vi "ReadWrite Channels.vi"(4 "ScheduledSDI":bool, 6 "Iteration":i32, 7 "Mode":T13, 8 "error in (no error)":errorcluster, 10 "FIFOs In":T14, 11 "Channels In":T1[](array[typedef]) {"Labels Settings"."Label" format="%.0o"}) -> (0 "error out":errorcluster, 2 "FIFOs Out":T14, 3 "Channels Out":T1[](array[typedef]) {"Labels Settings"."Label" format="%.0o"})   [LabVIEW 2015, in "AIT 429 Engine.lvlib"]
uses:
  AIT 429 Engine.lvlib
  RT Controls/FIFO.ctl
  RT Controls/ReadWrite Selector.ctl
  RT Controls/RT HW Channel.ctl
  RT Controls/RT Label Settings.ctl
  Shared/Controls and Global/Label.ctl
  Shared/Controls and Global/transferPeriod.ctl
  RT Controls/Driver Data.ctl
  RT Controls/RT Word Settings.ctl
  <vilib>/NI Veristand/Custom Device API/Block Data Reference.ctl
  <vilib>/NI Veristand/Custom Device API/Data Reference.ctl
  RT Controls/RT Param Setting.ctl
  Shared/Controls and Global/Start Bit.ctl
  Shared/Controls and Global/Number of Bits.ctl
  Shared/Controls and Global/TransferType.ctl
  Write outgoing label data.vi
  Read incoming label data.vi
  Read Parameter VS Channels.vi
  Update Parameter VS Channels.vi
  Double to selected bits.vi
  Shared/Word to double.vi
  <vilib>/NI Veristand/Custom Device API/NI VeriStand - Get Channel Values by Block Data Reference.vi
  <vilib>/NI Veristand/Custom Device API/NI VeriStand - Set Channel Values by Block Data Reference.vi
  <vilib>/NI Veristand/Custom Device API/Global Data Refs.vi
  <instrlib>/AIT 429/Public/Tx/Data/AIT 429 Set Acyclic Transfer Data.vi
  <instrlib>/AIT 429/Public/Tx/Data/AIT 429 Get Acyclic Transfer Data.vi
  <instrlib>/AIT 429/Public/Tx/Data/AIT 429 Set Block Transfer Data.vi
  <instrlib>/AIT 429/Public/Tx/Data/AIT 429 Get Block Transfer Data.vi
  <instrlib>/AIT 429/Public/Tx/Data/AIT 429 Set Scheduled Label Data.vi
  <instrlib>/AIT 429/Public/Tx/Data/AIT 429 Get Scheduled Label Data.vi
  <instrlib>/AIT 429/AIT 429.lvlib
  <userlib>/ARINC-429/Owl429.lvlib
  Shared/AIT 429 Shared.lvlib
  <vilib>/NI Veristand/Custom Device API/Custom Device API.lvlib
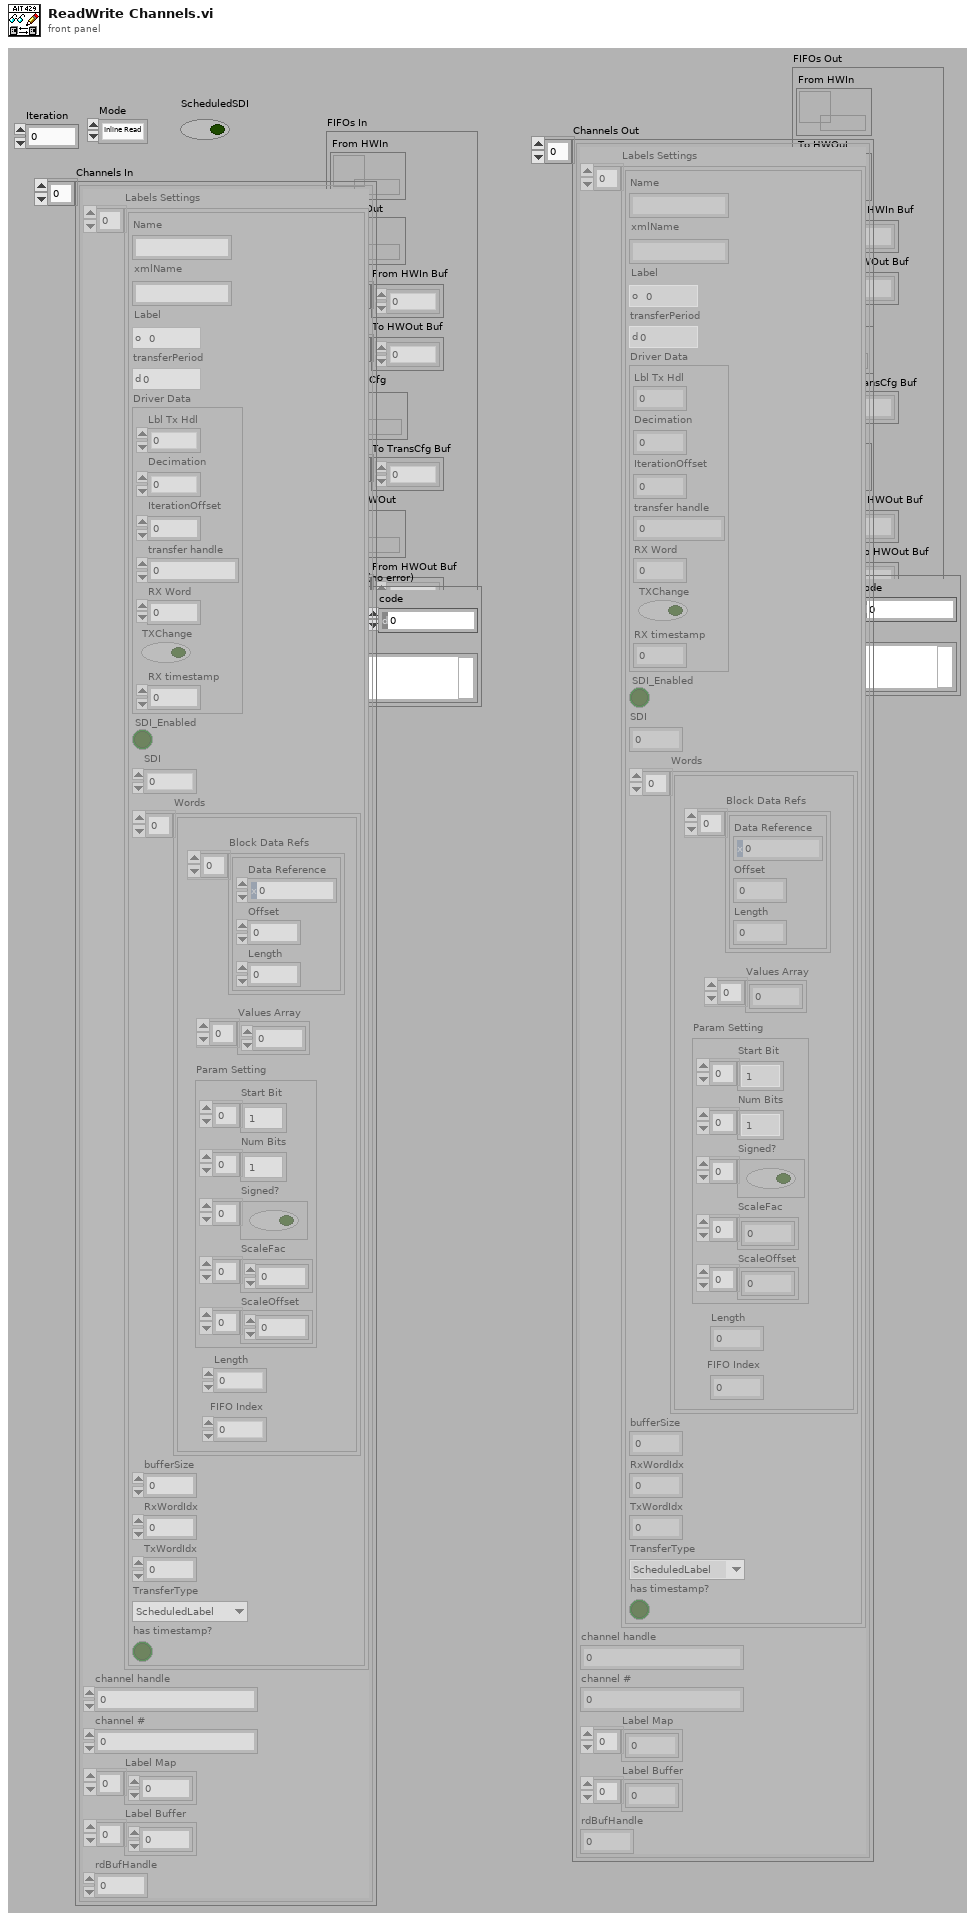
[diagram p1: front panel]
types:
  T1 = typedef "AIT 429 Engine.lvlib/RT HW Channel.ctl" = cluster{"Labels Settings":T2[], "channel handle":u32, "channel #":u16, "Label Map":i32[], "Label Buffer":u32[], "rdBufHandle":u32}
  T2 = typedef "AIT 429 Engine.lvlib/RT Label Settings.ctl" = cluster{"Name":string, "xmlName":string, "Label":T3, "transferPeriod":T4, "Driver Data":T5, "SDI_Enabled":bool, "SDI":u8, "Words":T6[], "bufferSize":u32, "RxWordIdx":i32, "TxWordIdx":i32, "TransferType":T12, "has timestamp?":bool}
  T3 = typedef "AIT 429 Shared.lvlib/Label.ctl" = u8
  T4 = typedef "AIT 429 Shared.lvlib/transferPeriod.ctl" = u32
  T5 = typedef "AIT 429 Engine.lvlib/Driver Data.ctl" = cluster{"Lbl Tx Hdl":u32, "Decimation":i32, "IterationOffset":i32, "transfer handle":u32, "RX Word":u32, "TXChange":bool, "RX timestamp":dbl}
  T6 = typedef "AIT 429 Engine.lvlib/RT Word Settings.ctl" = cluster{"Block Data Refs":T7[], "Values Array":dbl[], "Length":i32, "FIFO Index":i32, "Param Setting":T9}
  T7 = typedef "Custom Device API.lvlib/Block Data Reference.ctl" = cluster{"Data Reference":T8, "Offset":u64, "Length":u64}
  T8 = typedef "Custom Device API.lvlib/Data Reference.ctl" = i32
  T9 = typedef "AIT 429 Engine.lvlib/RT Param Setting.ctl" = cluster{"Start Bit":T10[], "Num Bits":T11[], "Signed?":bool[], "ScaleFac":dbl[], "ScaleOffset":dbl[]}
  T10 = typedef "AIT 429 Shared.lvlib/Start Bit.ctl" = i32
  T11 = typedef "AIT 429 Shared.lvlib/Number of Bits.ctl" = i32
  T12 = typedef "AIT 429 Shared.lvlib/TransferType.ctl" = enum16{"ScheduledLabel", "Acyclic", "Block", "Strobe"}
  T13 = typedef "AIT 429 Engine.lvlib/ReadWrite Selector.ctl" = enum16{"Inline Read", "Inline Write", "Async HWIn", "Async HWOut"}
  T14 = typedef "AIT 429 Engine.lvlib/FIFO.ctl" = cluster{"From HWIn":refnum<k33>, "To HWOut":refnum<k33>, "From HWIn Buf":dbl[], "To HWOut Buf":dbl[], "To TansCfg":refnum<k33>, "To TransCfg Buf":dbl[], "From HWOut":refnum<k33>, "From HWOut Buf":dbl[], "Old To HWOut Buf":dbl[]}
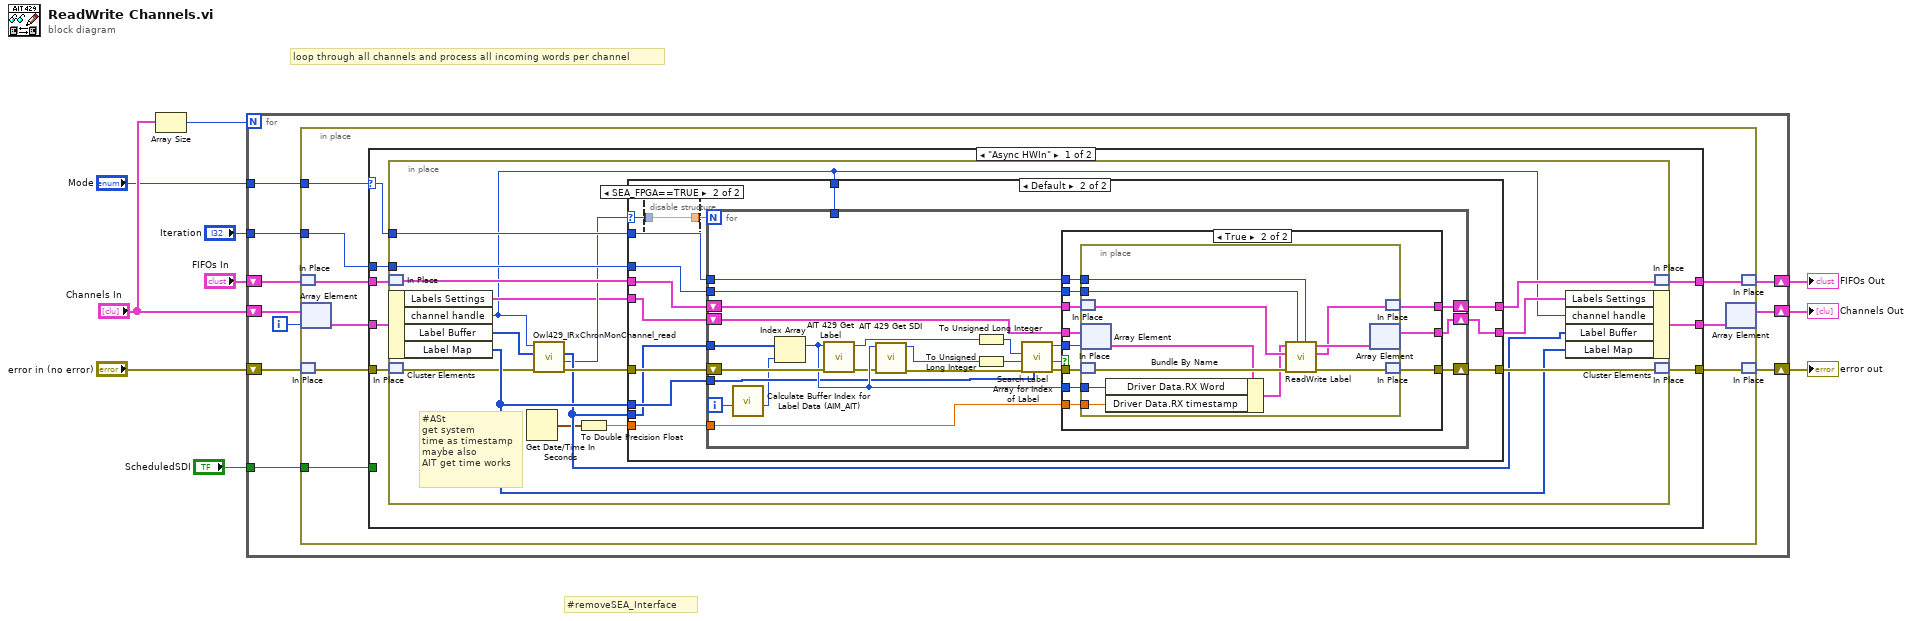
[diagram p0: block diagram]
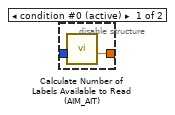
[diagram p3: hidden frame]
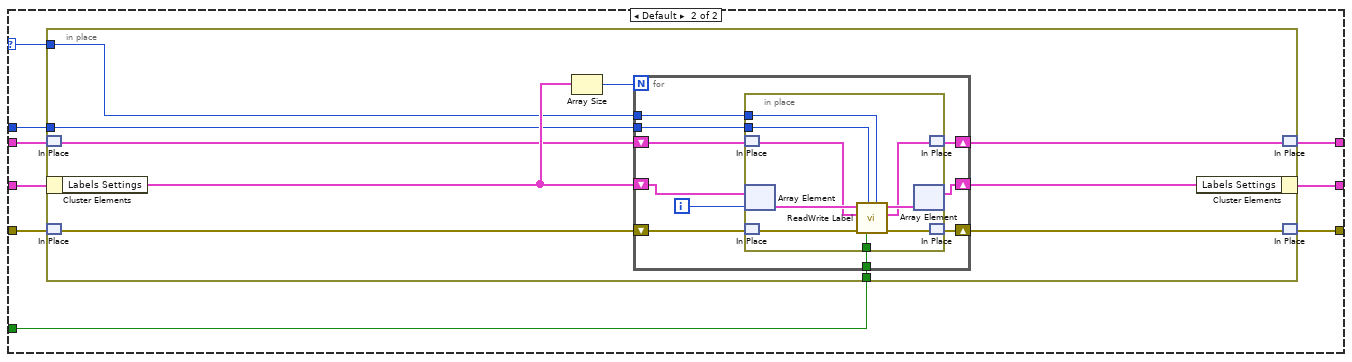
[diagram p5: hidden frame]
diagram:
  # "#removeSEA_Interface"
  # "loop through all channels and process all incoming words per channel"
  n1 = Array Size(array="Channels In") -> (size(s)=w5:i32)
  n2 = for {
    N: w5 -> [_]
    shift-right: [w17] -> w8
    shift-left: "error in (no error)" -> [w18]
    tunnel: "Mode" -> [w16]
    tunnel: "Iteration" -> [w13]
    shift-right: [w19] -> w7
    shift-left: "Channels In" -> [w20]
    shift-right: [w14] -> w10
    shift-left: "FIFOs In" -> [w15]
    tunnel: "ScheduledSDI" -> [w12]
    i -> [w11]
    n3 = in-place {
      in-place-border: w16 -> [w22]
      in-place-border: w13 -> [w23]
      in-place-border: w12 -> [w21]
      n4 = in-place-match #1(w15) -> (w25:T14)
      n5 = in-place-array #2(w20, w11) -> (w29:T1)
      n6 = in-place-match #3(w18) -> (w27:errorcluster)
      n7 = case shown="\"Async HWIn\"" w22 {
        selector: w22 -> [w30 w123]
        tunnel: w29 -> [w37 w130]
        tunnel: [w36 w129] -> w28
        tunnel: w27 -> [w35 w128]
        tunnel: [w34 w127] -> w26
        tunnel: w25 -> [w33 w126]
        tunnel: [w32 w125] -> w24
        tunnel: w23 -> [w31 w124]
        tunnel: w21 -> [_ w122]
        frame "Async HWIn" {
          n8 = in-place {
            in-place-border: w30 -> [w51]
            in-place-border: w31 -> [w49]
            # "#ASt\nget system\ntime as timestamp\nmaybe also\nAIT get time works"
            n9 = in-place-match #4(w33) -> (w48:T14)
            n10 = in-place-cluster #5(w37) -> ("Labels Settings"=w41:T2[], "channel handle"=w38:u32, "Label Buffer"=w42:u32[], "Label Map"=w47:i32[])
            n11 = in-place-match #6(w35) -> (w45:errorcluster)
            n12 = Get Date/Time In Seconds() -> (seconds since 1Jan1904=w40:timestamp)
            n13 = call <userlib>:"Owl429_IRxChronMonChannel_read.vi"("error in (no error)"=w45, "data buffer"=w42, "channel handle"=w38) -> ("error out"=w46:errorcluster, "word count"=w43:u32, "data buffer"=w44:u32[])  [unwired: 5 in, 1 out]
            n14 = To Double Precision Float(number=w40) -> (double precision float=w39:dbl)
            n15 = case shown="Default" w43 {
              selector: w43 -> [_ w59]
              tunnel: w41 -> [w55 w70]
              tunnel: [w55 w69] -> w53
              tunnel: [w56 w68] -> w52
              tunnel: w51 -> [_ w67]
              tunnel: [w54 w66] -> w50
              tunnel: w49 -> [_ w65]
              tunnel: w48 -> [w54 w64]
              tunnel: w47 -> [_ w63]
              tunnel: w46 -> [w56 w62]
              tunnel: w44 -> [_ w61]
              tunnel: w39 -> [_ w58]
              tunnel: w38 -> [_ w57]
              frame 0 {
              }
              frame Default {
                n16 = disable-structure shown="SEA_FPGA==TRUE" {
                  disable-tunnel: [w72 w73] -> w60
                  disable-tunnel: w59 -> [w71 w73]
                  frame condition #0 (active) {
                    n17 = call "Calculate Number of Labels Available to Read (AIM_AIT).vi"("entry count"=w71) -> ("# of labels available"=w72:dbl)  [unwired: 10 in]
                  }
                  frame condition #1 {
                  }
                }
                n18 = for {
                  N: w60 -> [_]
                  shift-right: [w95] -> w68
                  shift-left: w62 -> [w90]
                  tunnel: w67 -> [w94]
                  tunnel: w65 -> [w91]
                  tunnel: w61 -> [w86]
                  shift-right: [w92] -> w66
                  shift-left: w64 -> [w93]
                  shift-right: [w96] -> w69
                  shift-left: w70 -> [w89]
                  tunnel: w63 -> [w76]
                  tunnel: w58 -> [w77]
                  tunnel: w57 -> [_]
                  i -> [w84]
                  n19 = call "Calculate Buffer Index for Label Data (AIM_AIT).vi"("Iteration"=w84) -> ("Buffer index"=w75:u32)  [unwired: 10 in]
                  n20 = Index Array(array=w86, index=w75) -> (element=w80:u32)
                  n21 = call <instrlib>:"AIT 429 Get Label.vi"("error in (no error)"=w90, "word"=w80) -> ("error out"=w74:errorcluster, "label"=w81:u8)  [unwired: 8 in]
                  n22 = call <instrlib>:"AIT 429 Get SDI.vi"("error in (no error)"=w74, "word"=w80) -> ("error out"=w82:errorcluster, "sdi"=w83:u8)  [unwired: 8 in]
                  n23 = To Unsigned Long Integer(number=w81) -> (unsigned 32bit integer=w79:u32)
                  n24 = To Unsigned Long Integer(number=w83) -> (unsigned 32bit integer=w78:u32)
                  n25 = call "Search Label Array for Index of Label.vi"("Label Map"=w76, "error in (no error)"=w82, "sdi"=w78, "label"=w79) -> ("error out"=w87:errorcluster, "Label Found?"=w85:bool, "Index"=w88:i32)  [unwired: 5 in]
                  n26 = case shown="True" w85 {
                    tunnel: [w98 w110] -> w96
                    tunnel: [w97 w109] -> w95
                    tunnel: w94 -> [_ w108]
                    tunnel: w93 -> [w99 w107]
                    tunnel: [w99 w106] -> w92
                    tunnel: w91 -> [_ w105]
                    tunnel: w89 -> [w98 w104]
                    tunnel: w88 -> [_ w103]
                    tunnel: w87 -> [w97 w102]
                    tunnel: w80 -> [_ w101]
                    tunnel: w77 -> [_ w100]
                    frame False {
                    }
                    frame True {
                      n27 = in-place {
                        in-place-border: w108 -> [w118]
                        in-place-border: w105 -> [w117]
                        in-place-border: w101 -> [w112]
                        in-place-border: w100 -> [w111]
                        n28 = in-place-match #7(w107) -> (w116:T14)
                        n29 = in-place-array #8(w104, w103) -> (w114:T2)
                        n30 = in-place-match #9(w102) -> (w121:errorcluster)
                        n31 = Bundle By Name(cluster=w114, "Driver Data.RX Word"=w112, "Driver Data.RX timestamp"=w111) -> (w113:T2)
                        n32 = call "ReadWrite Label.vi"("Mode"=w118, "Iteration"=w117, "error in (no error)"=w121, "FIFOs In"=w116, "Label In"=w113) -> ("error out"=w120:errorcluster, "FIFOs Out"=w115:T14, "Label Out"=w119:T2)  [unwired: 4 in]
                        n33 = in-place-array #8(w119) -> (w110:T2[])  [unwired: 1 out]
                        n34 = in-place-match #7(w115) -> (w106:T14)
                        n35 = in-place-match #9(w120) -> (w109:errorcluster)
                      }
                    }
                  }
                }
              }
            }
            n36 = in-place-cluster #5("Labels Settings"=w53, "channel handle"=w38, "Label Buffer"=w44, "Label Map"=w47) -> (w36:T1)
            n37 = in-place-match #4(w50) -> (w32:T14)
            n38 = in-place-match #6(w52) -> (w34:errorcluster)
          }
        }
        frame Default {
          n39 = in-place {
            in-place-border: w123 -> [w136]
            in-place-border: w124 -> [w134]
            in-place-border: w122 -> [w131]
            n40 = in-place-match #10(w126) -> (w133:T14)
            n41 = in-place-cluster #11(w130) -> ("Labels Settings"=w139:T2[])
            n42 = in-place-match #12(w128) -> (w132:errorcluster)
            n43 = Array Size(array=w139) -> (size(s)=w140:i32)
            n44 = for {
              N: w140 -> [_]
              shift-right: [w146] -> w137
              shift-left: w132 -> [w147]
              tunnel: w136 -> [w145]
              tunnel: w134 -> [w142]
              shift-right: [w143] -> w135
              shift-left: w133 -> [w144]
              shift-right: [w148] -> w138
              shift-left: w139 -> [w150]
              tunnel: w131 -> [w141]
              i -> [w149]
              n45 = in-place {
                in-place-border: w145 -> [w156]
                in-place-border: w142 -> [w157]
                in-place-border: w141 -> [w151]
                n46 = in-place-match #13(w144) -> (w152:T14)
                n47 = in-place-array #14(w150, w149) -> (w153:T2)
                n48 = in-place-match #15(w147) -> (w154:errorcluster)
                n49 = call "ReadWrite Label.vi"("Mode"=w156, "ScheduledSDI"=w151, "Iteration"=w157, "error in (no error)"=w154, "FIFOs In"=w152, "Label In"=w153) -> ("error out"=w159:errorcluster, "FIFOs Out"=w155:T14, "Label Out"=w158:T2)  [unwired: 3 in]
                n50 = in-place-array #14(w158) -> (w148:T2[])  [unwired: 1 out]
                n51 = in-place-match #13(w155) -> (w143:T14)
                n52 = in-place-match #15(w159) -> (w146:errorcluster)
              }
            }
            n53 = in-place-cluster #11("Labels Settings"=w138) -> (w129:T1)
            n54 = in-place-match #10(w135) -> (w125:T14)
            n55 = in-place-match #12(w137) -> (w127:errorcluster)
          }
        }
      }
      n56 = in-place-array #2(w28) -> (w19:T1[])  [unwired: 1 out]
      n57 = in-place-match #1(w24) -> (w14:T14)
      n58 = in-place-match #3(w26) -> (w17:errorcluster)
    }
  }
  "FIFOs Out" <- w10
  "error out" <- w8
  "Channels Out" <- w7
